vi "Error Query.vi"(8 "error in (no error)":errorcluster, 11 "VISA resource name":refnum<visa-resource-name>) -> (0 "error out":errorcluster, 1 "Error Message":string, 2 "Error Code":i32[](array[numeric]), 3 "VISA resource name out":refnum<visa-resource-name>)   [LabVIEW 2013, in "Agilent 3446X Series.lvlib"]
doc: "Queries the instrument for any errors in the instrument's error queue. It will continue to read errors until all errors have been read from the instrument. Any errors will be returned in the <B>error out</B> control.\n\n<B>Note:</B>\nThis VI is called automatically by most driver VIs so it is not usually necessary to call this in an application."
uses:
  <instrlib>/Agilent 3446X Series/Agilent 3446X Series.lvlib
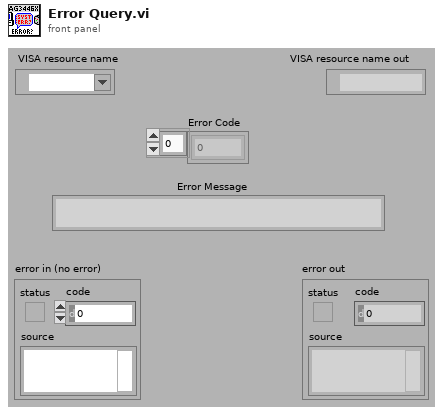
[diagram p1: front panel]
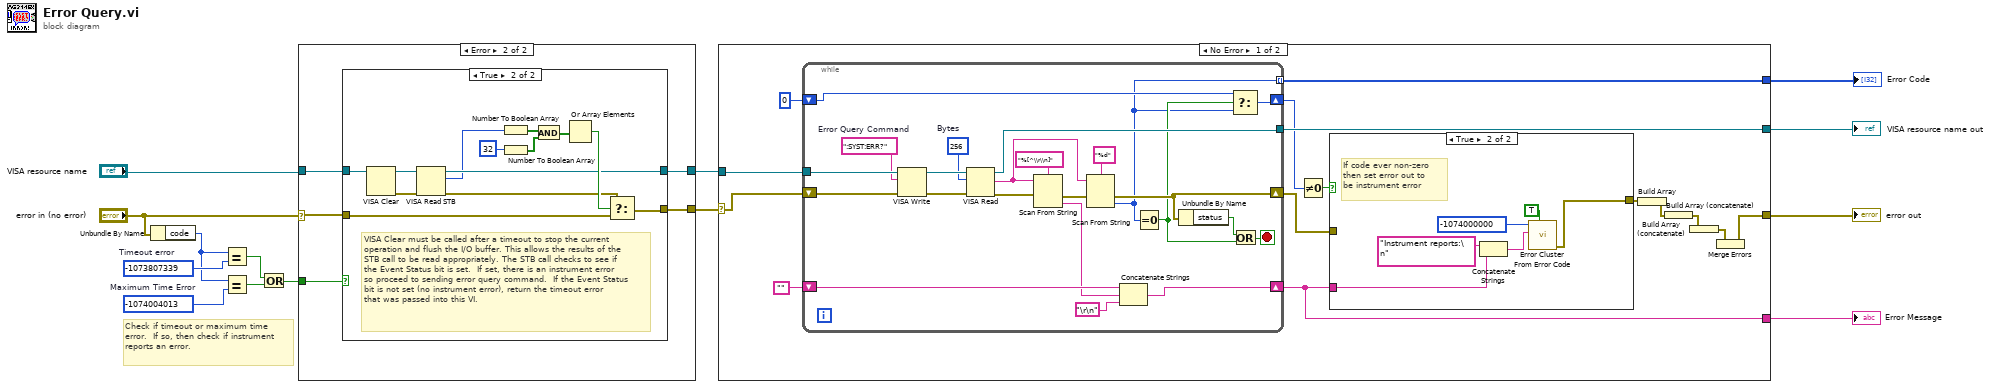
[diagram p0: block diagram]
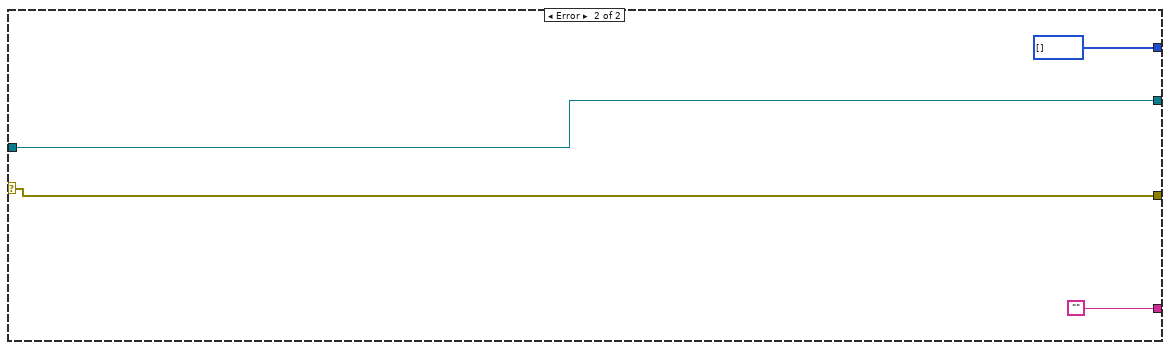
[diagram p5: hidden frame]
diagram:
  w5 = -1074004013  # Maximum Time Error
  w7 = -1073807339  # Timeout error
  # "Check if timeout or maximum time error.  If so, then check if instrument reports an error."
  n1 = Unbundle By Name("error in (no error)") -> ("code"=w6:i32)
  n2 = Equal?(x=w6, y=w7) -> (x = y?=w3:bool)
  n3 = Equal?(x=w6, y=w5) -> (x = y?=w4:bool)
  n4 = Or(x=w3, y=w4) -> (x .or. y?=w2:bool)
  n5 = case shown="Error" "error in (no error)" {
    selector: "error in (no error)" -> [w15 w19]
    tunnel: "VISA resource name" -> [w16 w21]
    tunnel: [w16 w20] -> w9
    tunnel: [w15 w18] -> w10
    tunnel: w2 -> [_ w17]
    frame No Error {
    }
    frame Error {
      n6 = case shown="True" w17 {
        tunnel: w21 -> [w23 w29]
        tunnel: [w23 w26] -> w20
        tunnel: w19 -> [w22 w32]
        tunnel: [w22 w31] -> w18
        frame False {
          # "Error code not a timeout, so best to pass on to user."
        }
        frame True {
          # "VISA Clear must be called after a timeout to stop the current operation and flush the I/O buffer. This allows the results of the  STB call to be read appropriately. The STB call checks to see if the Event Status bit is set.  If set, there is an instrument error so proceed to sending error query command.  If the Event Status bit is not set (no instrument error), return the timeout error that was passed into this VI."
          n7 = VISA Clear(VISA resource name=w29) -> (VISA resource name out=w28:refnum<visa-resource-name>, error out=w27:errorcluster)  [unwired: 1 in]
          n8 = VISA Read STB(8:w27, 11:w28) -> (0:w25:errorcluster, 2:w24:u16, 3:w26:refnum<visa-resource-name>)
          n9 = Number To Boolean Array(number=w24) -> (Boolean array=w33:bool[])
          n10 = Number To Boolean Array(number=32) -> (Boolean array=w35:bool[])
          n11 = And(x=w33, y=w35) -> (x .and. y?=w34:bool[])
          n12 = Or Array Elements(Boolean array=w34) -> (logical OR=w30:bool)
          n13 = Select(t=w25, s=w30, f=w32) -> (s? t:f=w31:errorcluster)
        }
      }
    }
  }
  n14 = case shown="No Error" w10 {
    selector: w10 -> [w40 w82]
    tunnel: [w51 w85] -> w14
    tunnel: w9 -> [w50 w85]
    tunnel: [w48 w82] -> w13
    tunnel: [w43 ""] -> w12
    tunnel: [w42 i32[] []] -> w11
    frame No Error {
      n15 = while {
        tunnel: [w81] -> w51
        tunnel: w50 -> [w80]
        shift-right: [w68] -> w43
        shift-left: "" -> [w71]
        shift-right: [w66] -> w44
        shift-left: 0 -> [w67]
        shift-right: [w64] -> w41
        shift-left: w40 -> [w65]
        tunnel: [w59] -> w42 mode=indexing
        stop <- w74 stop-if-true
        w78 = u32 256  # Bytes
        w76 = ":SYST:ERR?"  # Error Query Command
        n16 = VISA Write(VISA resource name=w80, write buffer=w76, error in (no error)=w65) -> (VISA resource name out=w79:refnum<visa-resource-name>, error out=w77:errorcluster)  [unwired: 1 out]
        n17 = VISA Read(VISA resource name=w79, byte count=w78, error in (no error)=w77) -> (VISA resource name out=w81:refnum<visa-resource-name>, read buffer=w72:string, error out=w63:errorcluster)  [unwired: 1 out]
        n18 = Scan From String(format string="%[^\\r\\n]", input string=w72, error in=w63) -> (error out=w62:errorcluster, output 1=w69:string)  [unwired: 1 in, 3 out]
        n19 = Scan From String(format string="%d", input string=w72, error in=w62) -> (error out=w64:errorcluster, output 1=w59:i32)  [unwired: 1 in, 3 out]
        n20 = Concatenate Strings(w71, w69, "\r\n") -> (w68:string)
        n21 = Equal To 0?(x=w59) -> (x = 0?=w60:bool)
        n22 = Unbundle By Name(w64) -> ("status"=w61:bool)
        n23 = Select(t=w67, s=w60, f=w59) -> (s? t:f=w66:i32)
        n24 = Or(x=w61, y=w60) -> (x .or. y?=w74:bool)
      }
      n25 = Not Equal To 0?(x=w44) -> (x != 0?=w46:bool)
      n26 = case shown="True" w46 {
        tunnel: w43 -> [_ w57]
        tunnel: [w52 w53] -> w45
        tunnel: w41 -> [w52 _]
        frame False {
        }
        frame True {
          # "If code ever non-zero\nthen set error out to\nbe instrument error"
          n27 = Concatenate Strings("Instrument reports:\n" ("Source"), w57) -> (w54:string)
          n28 = call <vilib>:"Error Cluster From Error Code.vi"("show call chain? (False)"=TRUE, "error message (\"\")"=w54, "error code (0)"=-1074000000 ("Code")) -> ("error out"=w53:errorcluster)  [unwired: 1 in, 5 out]
        }
      }
      n29 = Build Array(w45) -> (w39:errorcluster[])
      n30 = Build Array (concatenate)(w39) -> (w38:errorcluster[])
      n31 = Build Array (concatenate)(w38) -> (w37:errorcluster[])
      n32 = Merge Errors(w37) -> (w48:errorcluster)
    }
    frame Error {
    }
  }
  "VISA resource name out" <- w14
  "error out" <- w13
  "Error Message" <- w12
  "Error Code" <- w11
